vi "Render Ship.vi"(7 "Renderer":refnum<class "Renderer.lvclass">, 8 "error in (no error)":errorcluster, 10 "Camera":refnum<class "Camera.lvclass">, 11 "Slylandro in":refnum<class "Slylandro.lvclass">) -> (0 "error out":errorcluster)   [LabVIEW 2021, in "Slylandro.lvclass"]
uses:
  Slylandro.lvclass
  Camera/Camera.lvclass
  Renderer/Renderer.lvclass
  Slylandro.lvclass/Slylandro.ctl
  C:/dev/LabVIEW/LabMelee/Source/Application Specific/Ship/Ship.lvclass
  C:/dev/LabVIEW/LabMelee/Source/Application Specific/Element/Element.lvclass
  C:/dev/LabVIEW/LabMelee/Source/Application Specific/Ships/Slylandro/Slylandro.lvclass
  Motion/Motion.lvclass
  Element/Element.lvclass
  Resource Manager/Resource Manager.lvclass
  Vector 2D/Vector 2D.lvclass
  Ship/Ship.lvclass
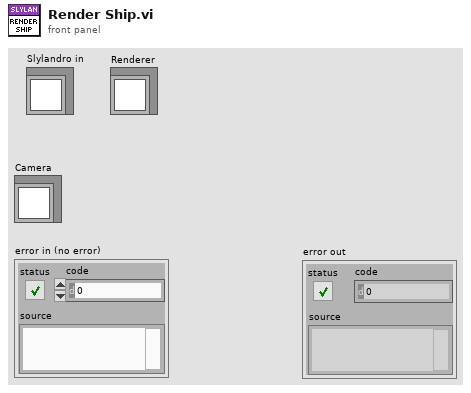
[diagram p1: front panel]
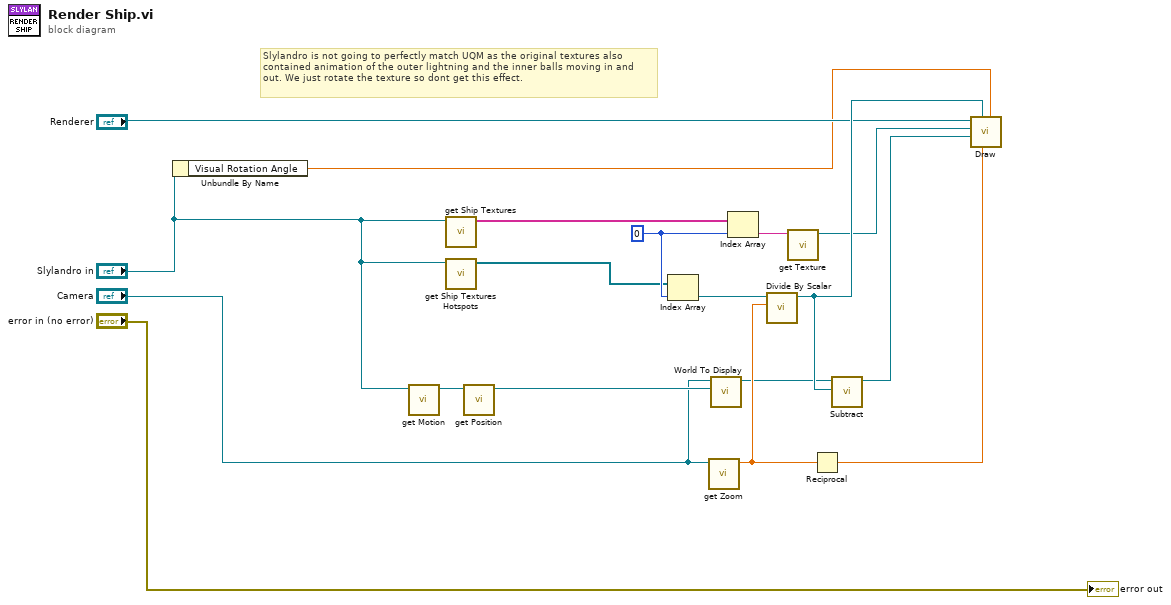
[diagram p0: block diagram]
diagram:
  w17 = 0 ("Texture Index")
  # "Slylandro is not going to perfectly match UQM as the original textures also contained animation of the outer lightning and the inner balls moving in and out. We just rotate the texture so dont get this effect."
  n1 = Unbundle By Name("Slylandro in") -> ("Visual Rotation Angle"=w1:dbl)
  n2 = call "get Motion.vi"("Element in"="Slylandro in") -> ("Motion"=w8:refnum<class "Motion.lvclass">)  [unwired: 10 in]
  n3 = call "get Ship Textures.vi"("Ship in"="Slylandro in") -> ("Ship"=w4:string[])  [unwired: 10 in]
  n4 = call "get Ship Textures Hotspots.vi"("Ship in"="Slylandro in") -> ("Ship Hotspots"=w3:refnum<class "Vector 2D.lvclass">[])  [unwired: 10 in]
  n5 = call "get Position.vi"("Motion in"=w8) -> ("Displacement"=w10:refnum<class "Vector 2D.lvclass">)  [unwired: 10 in]
  n6 = Index Array(array=w3, index=w17) -> (element=w14:refnum<class "Vector 2D.lvclass">)
  n7 = call "get Zoom.vi"("Camera in"="Camera") -> ("Zoom Level"=w15:sgl)  [unwired: 10 in]
  n8 = call "World To Display.vi"("World Position"=w10, "Camera in"="Camera") -> ("Display Position"=w13:refnum<class "Vector 2D.lvclass">)  [unwired: 9 in]
  n9 = Index Array(array=w4, index=w17) -> (element=w9:string)
  n10 = call "Divide By Scalar.vi"("x"=w15, "A"=w14) -> ("Ax"=w18:refnum<class "Vector 2D.lvclass">)  [unwired: 9 in]
  n11 = call "get Texture.vi"("Texture Name"=w9) -> ("Texture"=w12:refnum<class "Texture.lvclass">)  [unwired: 10 in]
  n12 = Reciprocal(x=w15) -> (1/x=w11:sgl)
  n13 = call "Subtract.vi"("B"=w18, "A"=w13) -> ("A-B"=w16:refnum<class "Vector 2D.lvclass">)  [unwired: 9 in]
  n14 = call "Draw.vi"("Angle"=w1, "Scale"=w11, "Rotation Center"=w18, "Destination"=w16, "Texture"=w12, "Renderer"="Renderer") -> ()  [unwired: 5 in, 1 out]
  "error out" <- "error in (no error)"
